vi "Command+Time String Loop.vi"() -> ()   [LabVIEW 2019, in "Part of Main VIs.lvlib" / "Command Library.lvlib"]
uses:
  Command Library.lvlib
  110c7450-e510-4401-b30d-b616388d447d.vi
  <extravilib>/ChannelInstances/Tag-bool/Read With Abort.vi
  <extravilib>/ChannelInstances/Tag-str/Write With Abort.vi
  <extravilib>/ChannelInstances/Tag-bool/Write With Abort.vi
  <extravilib>/ChannelInstances/Tag-str/Read With Abort.vi
  <extravilib>/ChannelInstances/Tag-bool/Instantiate.vi
  <extravilib>/ChannelInstances/Tag-str/Instantiate.vi
  <extravilib>/ChannelInstances/Tag-bool/Endpoint.vi
  <extravilib>/ChannelInstances/Tag-str/EndpointRead.vi
  <extravilib>/ChannelInstances/Tag-bool/EndpointRead.vi
  <extravilib>/ChannelInstances/Tag-str/Endpoint.vi
  <extravilib>/ChannelInstances/Tag-str.lvlib
  Command VI.lvlib
  <extravilib>/ChannelInstances/Tag-bool.lvlib
panel:
  out "error out":errorcluster
  out "path":path
  in  "String":string
  in  "stop":bool
  out "Command History":string
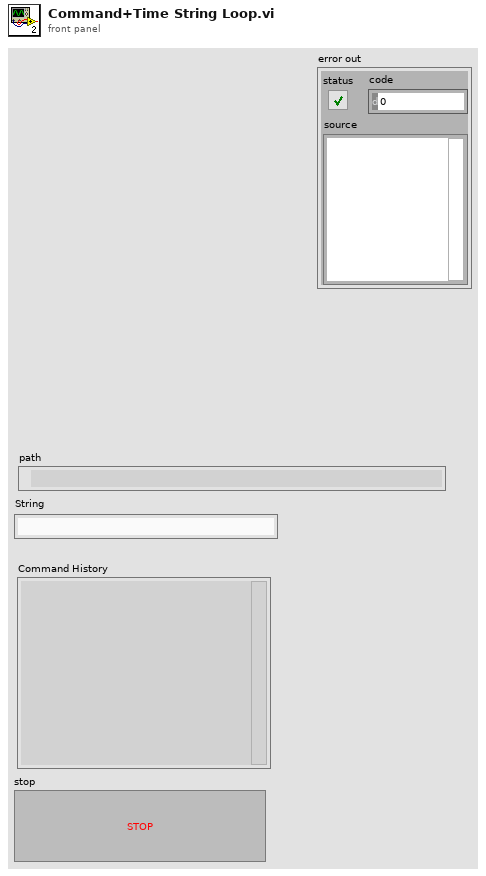
[diagram p1: front panel]
types:
  T1 = enum16{"open", "replace", "create", "open or create", "replace or create", "replace or create with confirmation"}
  T2 = typedef "Tag-bool.lvlib/))Channel.ctl" = refnum<queue>
  T3 = typedef "Tag-str.lvlib/))Channel.ctl" = refnum<queue>
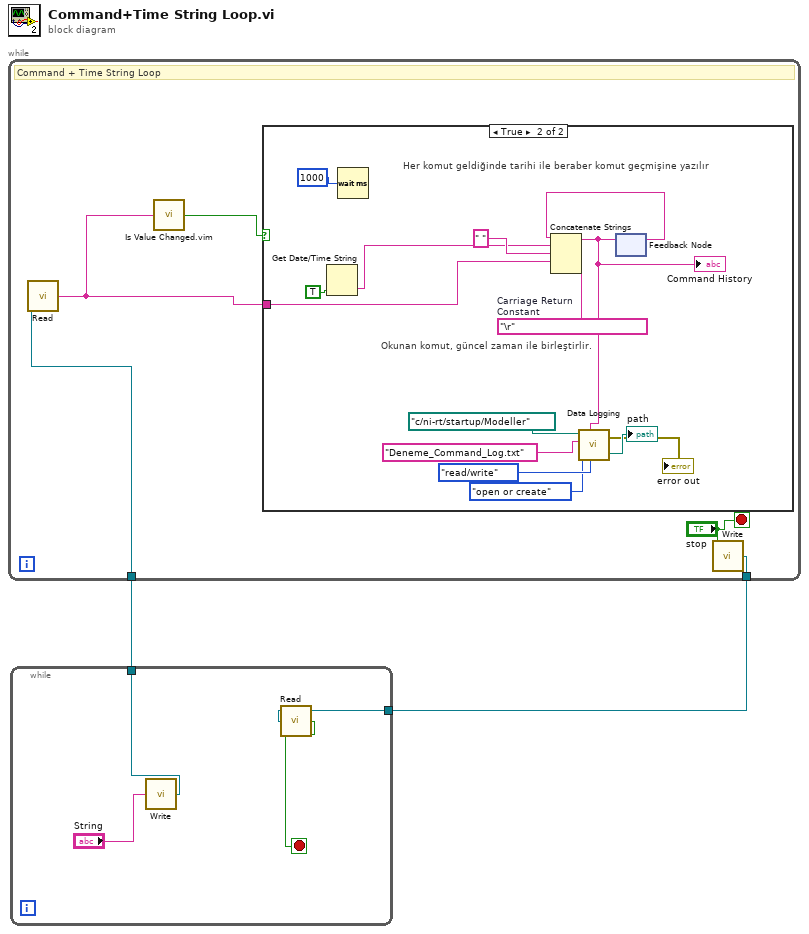
[diagram p0: block diagram]
diagram:
  n1 = while {
    tunnel: w2 -> [w6]
    tunnel: [w3] -> w1
    stop <- "stop" stop-if-true
    # "Command + Time String Loop"
    n2 = call <extravilib>:"Read.vi"("channel"=w6) -> ("element"=w4:string)  [unwired: 1 in, 1 out]
    n3 = call "Is Value Changed.vim"("value"=w4) -> ("changed or first call?"=w5:bool)
    n4 = case shown="True" w5 {
      tunnel: w4 -> [_ w21]
      frame False {
      }
      frame True {
        w18 = "\r"  # Carriage Return Constant
        # "Her komut geldiğinde tarihi ile beraber komut geçmişine yazılır"
        # "Okunan komut, güncel zaman ile birleştirlir."
        n5 = Get Date/Time String(want seconds? (F)=TRUE) -> (time string=w16:string)  [unwired: 2 in, 1 out]
        n6 = Wait (ms)(milliseconds to wait=u32 1000) -> ()  [unwired: 1 out]
        n7 = feedback #1() -> (w9:string)  [unwired: 1 in]
        n8 = Concatenate Strings "Concatenate Strings"(w9, w16, " " ("string"), w21, w18) -> (w8:string)
        "Command History" <- w8
        n9 = call "Data Logging.vi"("text"=w8, "access (0:read/write)"=enum16{"read/write", "read-only", "write-only"}."read/write", "operation (0:open)"=T1."open or create", "file"="Deneme_Command_Log.txt", "path"=path "c:/ni-rt/startup/Modeller") -> ("path"=→"path":path, "error out"=→"error out":errorcluster)  [unwired: 1 in]
        n10 = feedback-in #1(w8) -> ()
      }
    }
    n11 = call <extravilib>:"Write.vi"("element"="stop") -> ("channel"=w3:T2)  [unwired: 1 out]
  }
  n12 = while {
    tunnel: [w24] -> w2
    tunnel: w1 -> [w23]
    stop <- w22 stop-if-true
    n13 = call <extravilib>:"Write.vi"("element"="String") -> ("channel"=w24:T3)  [unwired: 1 out]
    n14 = call <extravilib>:"Read.vi"("channel"=w23) -> ("element"=w22:bool)  [unwired: 1 in, 1 out]
  }
